vi "Close Instrument.vi"(8 "error in (no error)":errorcluster, 11 "instrument.PPMS in":refnum<class "instrument.PPMS3.lvclass">) -> (0 "error out":errorcluster, 3 "instrument.PPMS out":refnum<class "instrument.PPMS3.lvclass">)   [LabVIEW 2016, in "instrument.PPMS3.lvclass"]
uses:
  instrument.PPMS3.lvclass
  instrument.PPMS3.lvclass/instrument.PPMS3.ctl
  C:/Users/patrick/Documents/GitHub/PPMS-Monitor-and-Control/lvsrc/drivers/QDInstrument_LabView/QDInstrument.dll
  drivers/QDInstrument_LabView/QDInstrument.dll
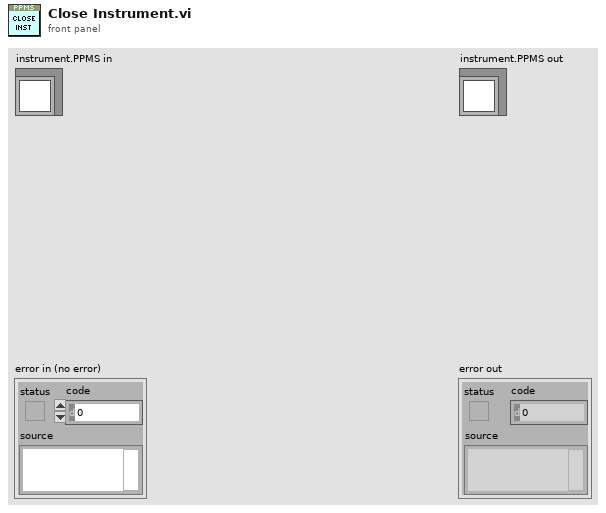
[diagram p1: front panel]
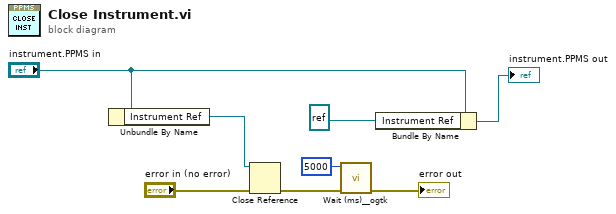
[diagram p0: block diagram]
diagram:
  n1 = Unbundle By Name("instrument.PPMS in") -> ("Instrument Ref"=w7:refnum<k24>)
  n2 = Close Reference(reference=w7, error in (no error)="error in (no error)") -> (error out=w3:errorcluster)
  n3 = call <userlib>:"Wait (ms)__ogtk.vi"("error in (no error)"=w3, "milliseconds to wait"=u32 5000) -> ("error out"=→"error out":errorcluster)  [unwired: 8 in, 1 out]
  n4 = Bundle By Name(cluster="instrument.PPMS in", "Instrument Ref"=refnum<k24> refnum) -> (→"instrument.PPMS out":refnum<class "instrument.PPMS3.lvclass">)
